vi "TCP Send with CRLF Dll.vi"(0 "CART TCP Connection":refnum<k5>, 7 "CommandIn":string) -> (4 "CART TCP Connection Out":refnum<k5>)   [LabVIEW 2011]
panel:
  in  "error IO":errorcluster
  out "error out":errorcluster
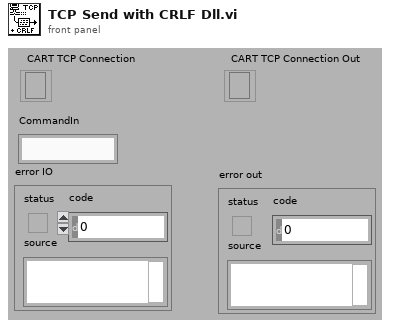
[diagram p1: front panel]
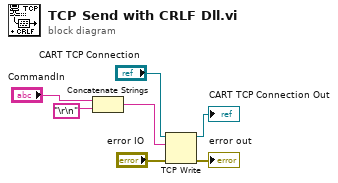
[diagram p0: block diagram]
diagram:
  n1 = Concatenate Strings("CommandIn", "\r\n") -> (w6:string)
  n2 = TCP Write(connection ID="CART TCP Connection", data in=w6, error in (no error)="error IO") -> (connection ID out=→"CART TCP Connection Out":refnum<k5>, error out=→"error out":errorcluster)  [unwired: 1 in, 1 out]
